vi "ingest.dataflash_free.vi"(8 "error in":errorcluster, 11 "DataflashIngestStaging in":refnum<class "DataflashIngestStaging.lvclass">) -> (0 "error out":errorcluster, 3 "DataflashIngestStaging out":refnum<class "DataflashIngestStaging.lvclass">)   [LabVIEW 2020, in "DataflashIngestStaging.lvclass"]
doc: "Releases the handle and its associated resources."
uses:
  DataflashIngestStaging.lvclass
  DataflashIngestStaging.lvclass/DataflashIngestStaging.ctl
  client.lvlib
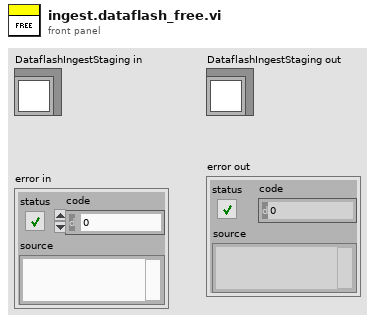
[diagram p1: front panel]
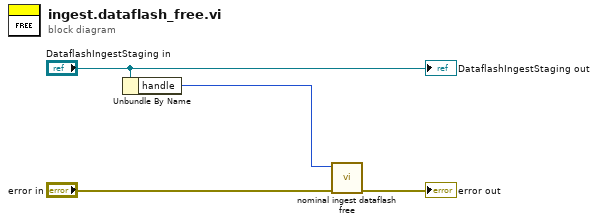
[diagram p0: block diagram]
diagram:
  n1 = Unbundle By Name("DataflashIngestStaging in") -> ("handle"=w2:i32)
  n2 = call "nominal ingest dataflash free.vi"("error in (no error)"="error in", "staging"=w2) -> ("error out"=→"error out":errorcluster)  [unwired: 8 in, 1 out]
  "DataflashIngestStaging out" <- "DataflashIngestStaging in"
